vi "Post_Process_Raw_data.vi"(0 "Select Plug Ins":bool, 2 "Post processed Results folder":path, 3 "No dialogs":bool, 5 "Save results to":T1(ring)=enum."Original Results Filenames with _PP", 11 "Selected files":path[](array[path]), 12 "Current Results filenames":path[](array[path]), 13 "Results Plotter Rows":string[][](array[string])) -> (15 "Post processed Results folder Out":path)   [LabVIEW 2014]
uses:
  Anemometry Sub Vis/Controls/File_Selector_Type.ctl
  Anemometry Sub Vis/Controls/Setup.ctl
  Anemometry Sub Vis/Controls/Post_Process.ctl
  Anemometry Sub Vis/Controls/Save_Data.ctl
  Anemometry Sub Vis/Globals/Meas_global.vi
  Anemometry Sub Vis/Data_plotting_vis/Results_plotter_Global.vi
  Anemometry Sub Vis/Globals/Plug_in_data_global.vi
panel:
  out "Single Filename":string
  out "Files not found":i32
  out "Files not Found":path[](array[path])
  out "Checking":i32
  in  "Previous Choice":path
  in  "Search String":string
  in  "Boolean":bool
  in  "Pause Mode":enum16{"Continuous Running", "After Each File"}(ring)
  in  "At Dialog Prompt Post Process":T2=enum."All files listed in selected file"
  out "Files Processed":i32(slide) scale=0.0..1.0
  in  "stop":bool
  out "Files To Process":path[](array[path])
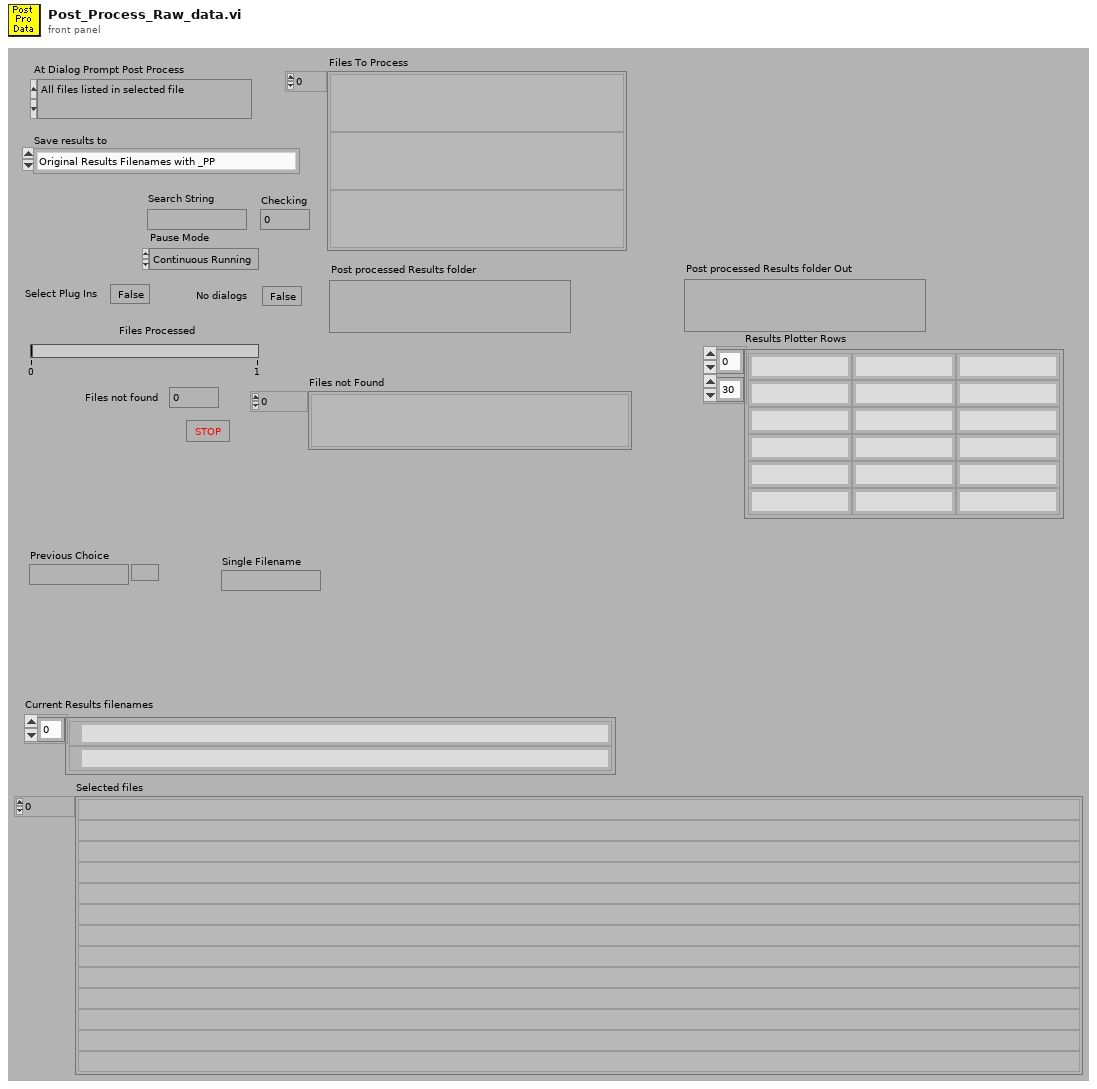
[diagram p1: front panel]
types:
  T1 = enum16{"A single file", "Original Results Filenames with _PP", "Current Results Filenames"}
  T2 = typedef "File_Selector_Type.ctl" = enum16{"The Selected File", "The Selected Folder", "Files containing the search string in the selected folder", "All files listed in selected file"}
  T3 = typedef "Setup.ctl" = enum16{"Run Program", "Show Setup", "Save Current Setup", "Setup Front Panel"}
  T4 = typedef "Save_Data.ctl" = enum16{"Save No Data", "Save Data"}
  T5 = typedef "Post_Process.ctl" = enum16{"Take New Data", "Post Process Raw Data File"}
  T6 = enum16{"Left Button", "Center Button", "Right Button", "Window Close"}
  T7 = typedef "Multi_Run_Status.ctl" = enum16{"Continue", "Jump to Next Point", "Jump to Next Row", "Jump To Fall Back", "Terminate Run"}
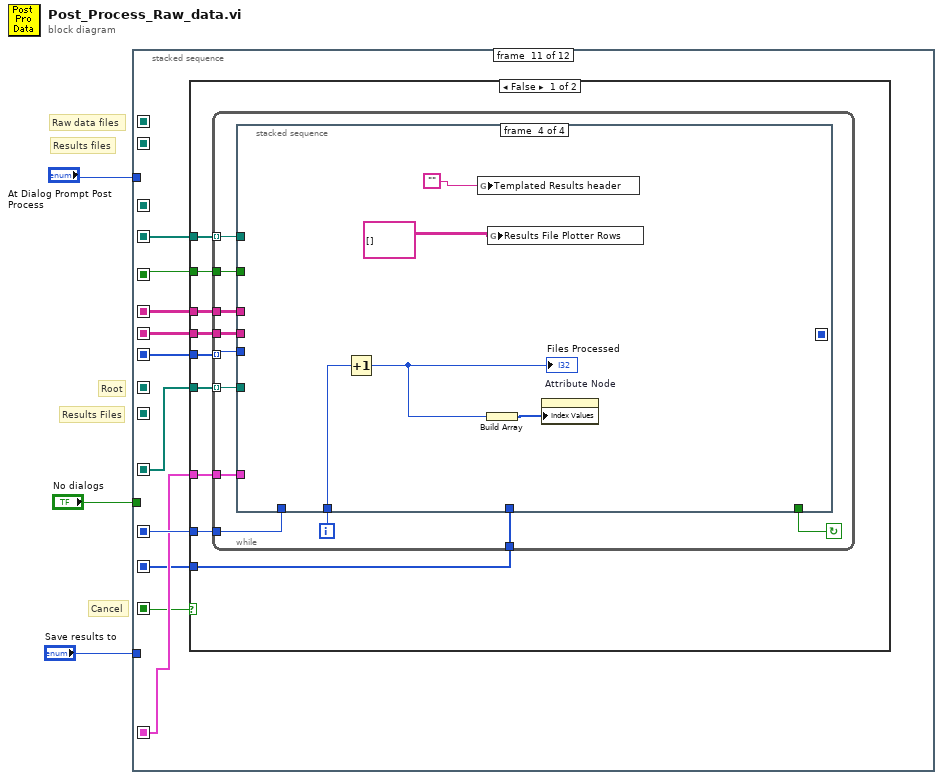
[diagram p0: block diagram]
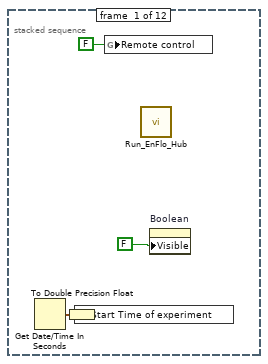
[diagram p2: hidden frame]
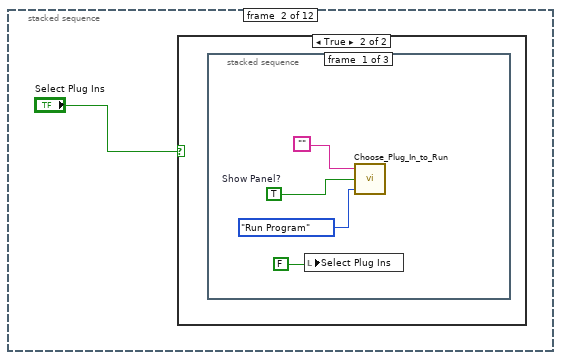
[diagram p3: hidden frame]
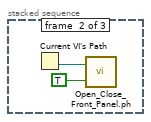
[diagram p5: hidden frame]
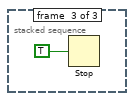
[diagram p6: hidden frame]
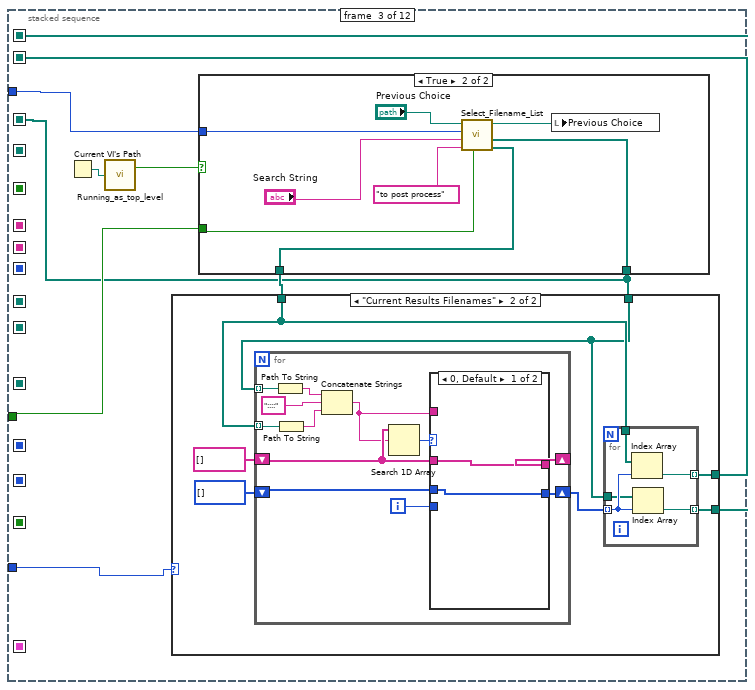
[diagram p7: hidden frame]
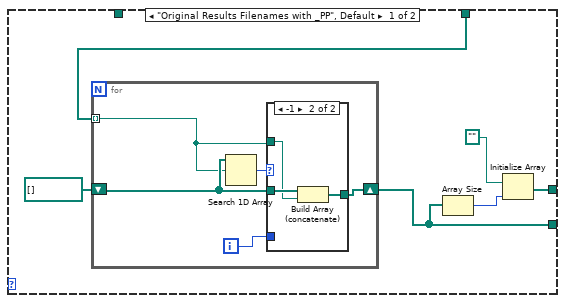
[diagram p8: hidden frame]
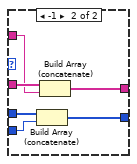
[diagram p10: hidden frame]
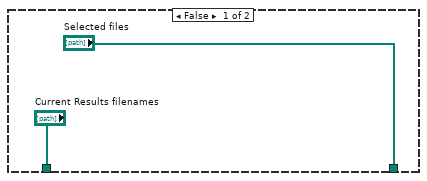
[diagram p11: hidden frame]
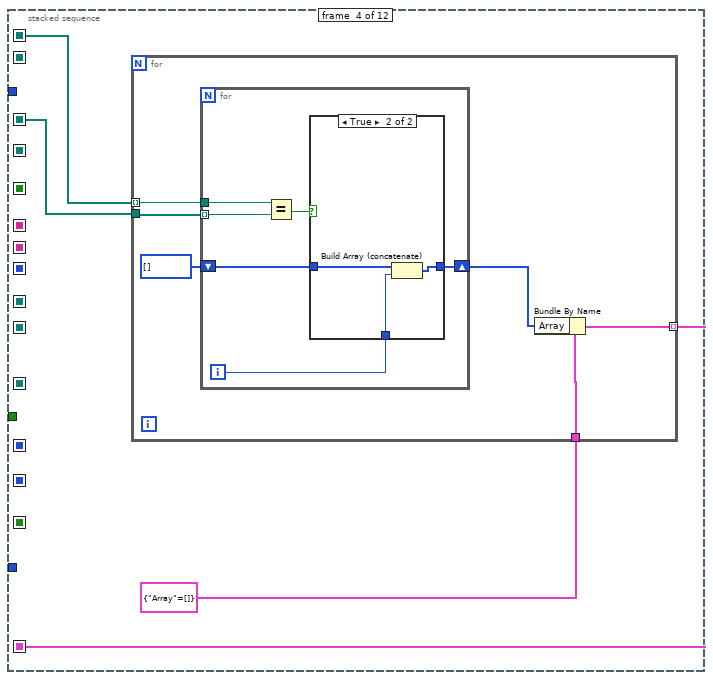
[diagram p12: hidden frame]
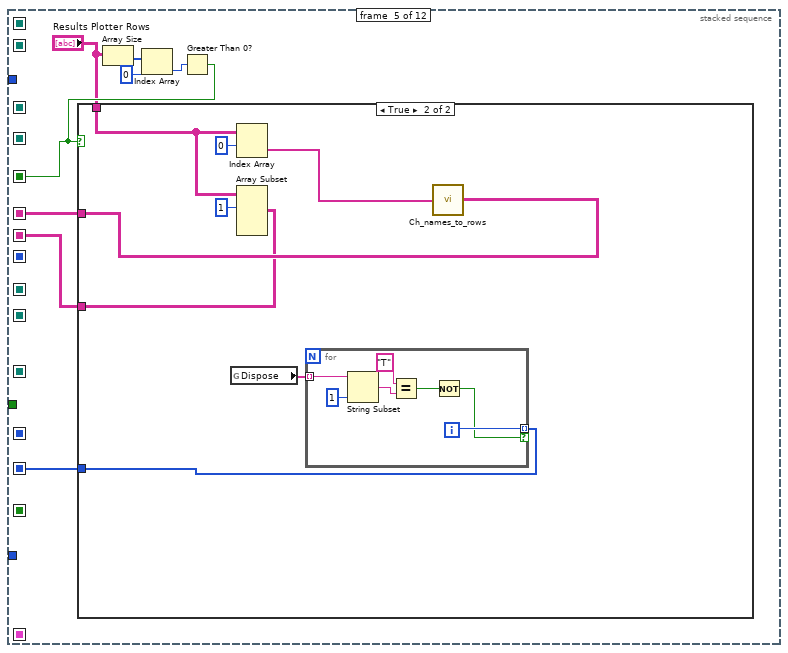
[diagram p14: hidden frame]
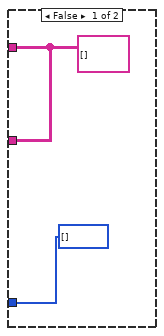
[diagram p15: hidden frame]
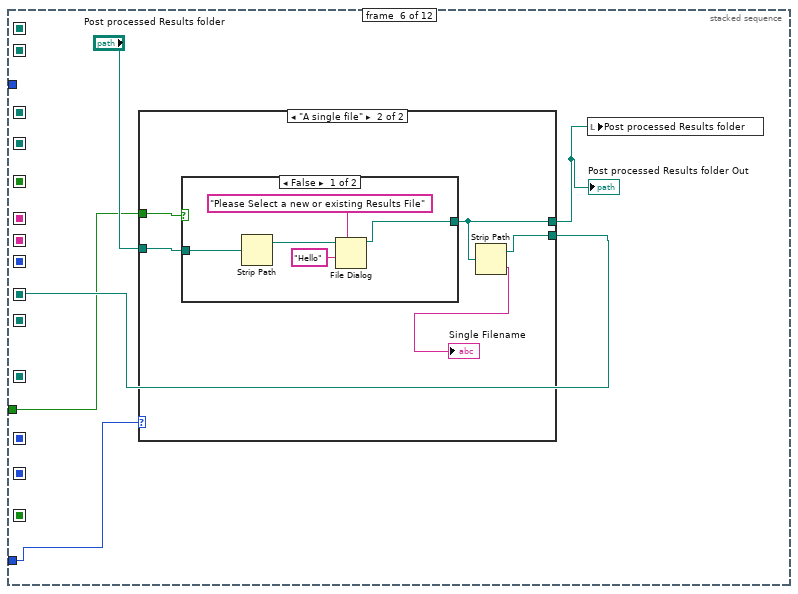
[diagram p16: hidden frame]
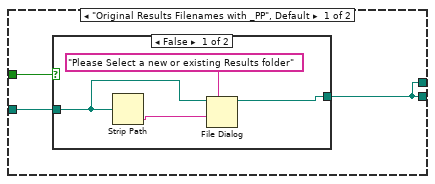
[diagram p17: hidden frame]
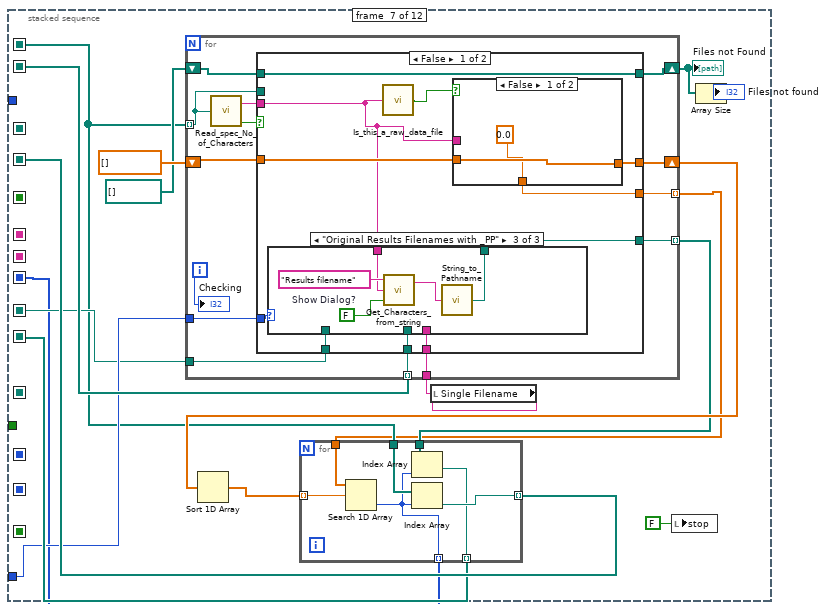
[diagram p20: hidden frame]
diagram:
  # "Cancel"
  # "Results files"
  # "Raw data files"
  # "Root"
  # "Results Files"
  n1 = stacked-sequence {
    seq-local: [_ _ _ _ _ _ w164 _ _ _ _ _] -> [_ _ _ _ _ _ _ _ _ w296 w311 _]
    seq-local: [_ _ _ _ _ _ _ _ _ w301 _ _] -> [_ _ _ _ _ _ _ _ _ _ w310 _]
    seq-local: [_ _ w18 _ _ _ _ _ _ _ _ _] -> [_ _ _ w84 _ _ w153 _ _ _ _ _]
    seq-local: [_ _ _ _ _ w131 _ _ _ _ _ _] -> [_ _ _ _ _ _ w156 w223 _ _ _ _]
    seq-local: [_ _ _ _ _ _ w162 _ _ _ _ _] -> [_ _ _ _ _ _ _ w226 _ _ _ _]
    seq-local: [_ _ _ _ _ _ _ w222 _ _ _ _] -> [_ _ _ _ _ _ _ _ w266 _ w309 w397]
    seq-local: [_ _ w19 _ _ _ _ _ _ _ _ _] -> [_ _ _ _ _ _ w158 _ _ _ _ _]
    seq-local: [_ _ _ _ w109 _ _ _ _ _ _ _] -> [_ _ _ _ _ _ _ _ _ _ w308 _]
    seq-local: [_ _ _ _ w108 _ _ _ _ _ _ _] -> [_ _ _ _ _ _ _ _ _ _ w305 _]
    seq-local: [_ _ _ _ w104 _ _ _ _ _ _ _] -> [_ _ _ _ _ _ _ _ _ _ w307 _]
    seq-local: [_ _ _ _ _ _ w154 _ _ _ _ _] -> [_ _ _ _ _ _ _ _ _ _ w306 _]
    seq-local: [_ _ _ w82 _ _ _ _ _ _ _ _] -> [_ _ _ _ _ _ _ _ _ _ w304 _]
    seq-local: [_ _ w16 _ _ _ _ _ _ _ _ _] -> [_ _ _ w85 _ _ _ _ _ _ _ _]
    seq-local: [_ _ _ _ _ _ _ _ w265 _ _ _] -> [_ _ _ _ _ _ _ _ _ _ w303 _]
    seq-local: [_ _ _ _ w102 _ _ _ _ _ _ _] -> [_ _ _ _ _ _ _ _ _ _ w302 _]
    tunnel: "At Dialog Prompt Post Process" -> [_ _ w24 _ _ _ _ _ _ _ _ _]
    tunnel: "No dialogs" -> [_ _ w23 _ _ w129 _ _ w267 _ _ _]
    tunnel: "Save results to" -> [_ _ w17 _ _ w128 w157 w225 _ _ _ _]
    frame #0 {
      n2 = Get Date/Time In Seconds() -> (seconds since 1Jan1904=w4:timestamp)
      n3 = To Double Precision Float(number=w4) -> (double precision float=w5:dbl)
      n4 = global write "Meas_global.vi" "Start Time of experiment"(w5) -> ()
      n5 = global write "Meas_global.vi" "Remote control"(FALSE ("Remote control")) -> ()
      n6 = call "Run_EnFlo_Hub.vi"() -> ()  [unwired: 8 out]
      n7 = property on="Boolean" class="Bool"("Visible"=FALSE ("Write Attribute")) -> ()  [unwired: 2 in, 2 out]
    }
    frame #1 {
      n8 = case shown="True" "Select Plug Ins" {
        frame False {
        }
        frame True {
          n9 = stacked-sequence {
            frame #0 {
              w12 = TRUE  # Show Panel?
              n10 = local write "Select Plug Ins"(FALSE ("Select Local ADAM Channels")) -> ()
              n11 = call "Choose_Plug_In_to_Run.vi"("setup"=Setup."Run Program", "Show Panel?"=w12, "Setup String In"="") -> ()  [unwired: 2 out]
            }
            frame #1 {
              n12 = Current VI's Path() -> (path=w14:path)
              n13 = call "Open_Close_Front_Panel.ph.vi"("Front Panel Window:Open"=TRUE, "VI path"=w14) -> ()  [unwired: 2 out]
            }
            frame #2 {
              n14 = Stop(stop? (T)=TRUE) -> ()
            }
          }
        }
      }
    }
    frame #2 {
      n15 = Current VI's Path() -> (path=w22:path)
      n16 = call "Running_as_top_level.vi"("Vi path name"=w22) -> ("Top Level"=w21:bool)  [unwired: 1 out]
      n17 = case shown="True" w21 {
        tunnel: w24 -> [_ w81]
        tunnel: w23 -> [_ w76]
        tunnel: ["Selected files" w75] -> w16
        tunnel: ["Current Results filenames" w74] -> w20
        frame False {
        }
        frame True {
          n18 = call "Select_Filename_List.vi"("No dialogs"=w76, "File Type"="to post process", "Search String"="Search String", "At Dialog Prompt Post Process"=w81, "Previous Choice"="Previous Choice") -> ("Current Results filenames"=w74:path[], "Selected files"=w75:path[], "Choosen path"=w77:path)  [unwired: 1 out]
          n19 = local write "Previous Choice"(w77) -> ()
        }
      }
      n20 = case shown="\"Current Results Filenames\"" w17 {
        tunnel: w16 -> [w30 w43]
        tunnel: w20 -> [_ w44]
        tunnel: [w26 w42] -> w19
        tunnel: [w28 w41] -> w18
        frame "Original Results Filenames with _PP", Default {
          n21 = for {
            shift-right: [w34] -> w28
            shift-left: path[] [] -> [w35]
            tunnel: w30 -> [w31] mode=indexing
            i -> [w32]
            n22 = Search 1D Array(1D array=w35, element=w31) -> (index of element=w33:i32)  [unwired: 1 out]
            n23 = case shown="-1" w33 {
              tunnel: w35 -> [w36 w39]
              tunnel: [w36 w38] -> w34
              tunnel: w31 -> [_ w37]
              tunnel: w32 -> [_ _]
              frame 0, Default {
              }
              frame -1 {
                n24 = Build Array (concatenate)(w39, w37) -> (w38:path[])
              }
            }
          }
          n25 = Array Size(array=w28) -> (size(s)=w27:i32)
          n26 = Initialize Array(path "", w27) -> (w26:path[])
        }
        frame "Current Results Filenames" {
          n27 = for {
            shift-right: [w62] -> _
            shift-left: string[] [] -> [w63]
            tunnel: w43 -> [w61] mode=indexing
            tunnel: w44 -> [w55] mode=indexing
            shift-right: [w57] -> w40
            shift-left: i32[] [] -> [w56]
            i -> [w58]
            n28 = Path To String(path=w61) -> (string=w60:string)
            n29 = Path To String(path=w55) -> (string=w54:string)
            n30 = Concatenate Strings(w60, "::::" ("string"), w54) -> (w53:string)
            n31 = Search 1D Array(1D array=w63, element=w53) -> (index of element=w52:i32)  [unwired: 1 out]
            n32 = case shown="0, Default" w52 {
              tunnel: w63 -> [w65 w71]
              tunnel: [w65 w70] -> w62
              tunnel: w53 -> [_ w67]
              tunnel: w58 -> [_ w66]
              tunnel: [w64 w69] -> w57
              tunnel: w56 -> [w64 w68]
              frame 0, Default {
              }
              frame -1 {
                n33 = Build Array (concatenate)(w68, w66) -> (w69:i32[])
                n34 = Build Array (concatenate)(w71, w67) -> (w70:string[])
              }
            }
          }
          n35 = for {
            tunnel: w40 -> [w51] mode=indexing
            tunnel: w44 -> [w50]
            tunnel: w43 -> [w49]
            tunnel: [w48] -> w42 mode=indexing
            tunnel: [w47] -> w41 mode=indexing
            n36 = Index Array(array=w50, index=w51) -> (element=w48:path)
            n37 = Index Array(array=w49, index=w51) -> (element=w47:path)
          }
        }
      }
    }
    frame #3 {
      n38 = for {
        tunnel: w85 -> [w90]
        tunnel: w84 -> [w91] mode=indexing
        tunnel: cluster{"Array":i64[]} {"Array"=[]} ("Cluster") -> [w88]
        tunnel: [w86] -> w82 mode=indexing
        n39 = for {
          tunnel: w91 -> [w97]
          tunnel: w90 -> [w96] mode=indexing
          shift-right: [w93] -> w87
          shift-left: i32[] [] -> [w94]
          i -> [w92]
          n40 = Equal?(x=w97, y=w96) -> (x = y?=w95:bool)
          n41 = case shown="True" w95 {
            tunnel: w94 -> [w98 w101]
            tunnel: [w98 w100] -> w93
            tunnel: w92 -> [_ w99]
            frame False {
            }
            frame True {
              n42 = Build Array (concatenate)(w101, w99) -> (w100:i32[])
            }
          }
        }
        n43 = Bundle By Name(cluster=w88, "Array"=w87) -> (w86:cluster{"Array":i64[]})
      }
    }
    frame #4 {
      n44 = Array Size(array="Results Plotter Rows") -> (size(s)=w107:i32[])
      n45 = Index Array(array=w107, index=0) -> (element=w105:i32)
      n46 = Greater Than 0?(x=w105) -> (x > 0?=w104:bool)
      n47 = case shown="True" w104 {
        tunnel: [w111 w119] -> w109
        tunnel: [w111 w114] -> w108
        tunnel: "Results Plotter Rows" -> [_ w117]
        tunnel: [i32[] [] w112] -> w102
        frame False {
          w111 = string[][] [] ("3 Row names")
        }
        frame True {
          n48 = global read "Results_plotter_Global.vi" "Dispose"() -> (w113:string[])
          n49 = Index Array(array=w117, index (row)=0 ("index")) -> (element=w115:string[])  [unwired: 1 in]
          n50 = Array Subset(array=w117, index (row)=1 ("index")) -> (w114:string[][])  [unwired: 3 in]
          n51 = for {
            tunnel: w113 -> [w123] mode=indexing
            tunnel: [w122] -> w112 mode=indexing if=w120
            i -> [w122]
            n52 = String Subset(string=w123, length (rest)=1 ("length (rest)")) -> (substring=w125:string)  [unwired: 1 out]
            n53 = Equal?(x="T", y=w125) -> (x = y?=w121:bool)
            n54 = Not(x=w121) -> (.not. x?=w120:bool)
          }
          n55 = call "Ch_names_to_rows.vi"("Channel Names"=w115) -> ("3 Row names"=w119:string[][])
        }
      }
    }
    frame #5 {
      n56 = case shown="\"A single file\"" w128 {
        tunnel: [w132 w141] -> w131
        tunnel: "Post processed Results folder" -> [w134 w144]
        tunnel: w129 -> [w133 w143]
        tunnel: [w132 w142] -> w127
        frame "Original Results Filenames with _PP", Default {
          n57 = case shown="False" w133 {
            tunnel: [w138 w139] -> w132
            tunnel: w134 -> [w135 w139]
            frame False {
              n58 = Strip Path(path=w135) -> (name=w136:string)  [unwired: 1 out]
              n59 = File Dialog(7:"Please Select a new or existing Results folder" ("prompt"), 9:w136, 11:w135) -> (3:w138:path)  [unwired: 1 in, 6 out]
            }
            frame True {
            }
          }
        }
        frame "A single file" {
          n60 = case shown="False" w143 {
            tunnel: w144 -> [w148 w150]
            tunnel: [w147 w150] -> w142
            frame False {
              n61 = Strip Path(path=w148) -> (stripped path=w146:path)  [unwired: 1 out]
              n62 = File Dialog(7:"Please Select a new or existing Results File" ("prompt"), 9:"Hello" ("default name"), 11:w146) -> (3:w147:path)  [unwired: 1 in, 6 out]
            }
            frame True {
            }
          }
          n63 = Strip Path(path=w142) -> (stripped path=w141:path, name=→"Single Filename":string)
        }
      }
      "Post processed Results folder Out" <- w127
      n64 = local write "Post processed Results folder"(w127) -> ()
    }
    frame #6 {
      n65 = local read "Single Filename"() -> (w155:string)
      n66 = for {
        tunnel: w153 -> [w183] mode=indexing
        shift-right: [w187] -> w167
        shift-left: dbl[] [] -> [w188]
        shift-right: [w184] -> w160
        shift-left: path[] [] -> [w185]
        tunnel: w158 -> [w180] mode=indexing
        tunnel: w157 -> [w179]
        tunnel: w156 -> [w178]
        tunnel: w155 -> [w177]
        tunnel: [w176] -> w152 mode=indexing
        tunnel: [w175] -> w151 mode=indexing
        i -> [w186]
        n67 = call "Read_spec_No_of_Characters.vi"("Filename"=w183) -> ("character string"=w182:string, "Error?"=w181:bool)
        n68 = case shown="False" w181 {
          tunnel: w188 -> [w199 w221]
          tunnel: [w198 w221] -> w187
          tunnel: w183 -> [_ w219]
          tunnel: w185 -> [w196 w220]
          tunnel: [w196 w218] -> w184
          tunnel: w182 -> [w195 _]
          tunnel: w180 -> [w193 w217]
          tunnel: w179 -> [w194 _]
          tunnel: w178 -> [w192 _]
          tunnel: w177 -> [w191 _]
          tunnel: [w190 w217] -> w176
          tunnel: [w189 0.0 ("Value")] -> w175
          frame False {
            n69 = case shown="\"Original Results Filenames with _PP\"" w194 {
              tunnel: [w202 w203 w206] -> w190
              tunnel: w195 -> [_ _ w204]
              tunnel: w193 -> [_ w203 _]
              tunnel: w192 -> [w201 _ _]
              tunnel: w191 -> [w200 _ _]
              frame "A single file" {
                n70 = Build Path(base path=w201, name or relative path=w200) -> (appended path=w202:path)
              }
              frame "Current Results Filenames" {
              }
              frame "Original Results Filenames with _PP" {
                w207 = FALSE  # Show Dialog?
                n71 = call "Get_Characters_from_string.vi"("Show Dialog?"=w207, "Input string"=w204, "Variable name"="Results filename") -> ("Value"=w205:string)  [unwired: 1 out]
                n72 = call "String_to_Pathname.vi"("Input String"=w205) -> ("path"=w206:path)
              }
            }
            n73 = call "Is_this_a_raw_data_file.vi"("character string"=w195) -> ("Raw Dat File?"=w197:bool)  [unwired: 2 out]
            n74 = case shown="False" w197 {
              tunnel: w199 -> [w210 w212]
              tunnel: [w210 w215] -> w198
              tunnel: w195 -> [_ w213]
              tunnel: [0.0 ("Value") w211] -> w189
              frame False {
              }
              frame True {
                n75 = call "Get_value_from_string.vi"("Input string"=w213, "Variable name"="Seconds since 1/1/04") -> ("Value"=w211:dbl)  [unwired: 1 in, 1 out]
                n76 = Build Array (concatenate)(w212, w211) -> (w215:dbl[])
              }
            }
          }
          frame True {
            n77 = Build Array (concatenate)(w220, w219) -> (w218:path[])
          }
        }
        "Checking" <- w186
      }
      "Files not Found" <- w160
      n78 = Sort 1D Array(array=w167) -> (sorted array=w166:dbl[])
      n79 = for {
        tunnel: w151 -> [w174]
        tunnel: w166 -> [w173] mode=indexing
        tunnel: w153 -> [w172]
        tunnel: [w171] -> w164 mode=indexing
        tunnel: w152 -> [w170]
        tunnel: [w169] -> w162 mode=indexing
        tunnel: [w168] -> w154 mode=indexing
        n80 = Search 1D Array(1D array=w174, element=w173) -> (index of element=w168:i32)  [unwired: 1 out]
        n81 = Index Array(array=w170, index=w168) -> (element=w169:path)
        n82 = Index Array(array=w172, index=w168) -> (element=w171:path)
      }
      n83 = local write "stop"(FALSE ("stop")) -> ()
      n84 = Array Size(array=w160) -> (size(s)=→"Files not found":i32)
    }
    frame #7 {
      n85 = case shown="\"Original Results Filenames with _PP\"" w225 {
        tunnel: [FALSE TRUE] -> w224
        tunnel: w225 -> [_ _]
        frame "A single file", Default {
        }
        frame "Original Results Filenames with _PP" {
        }
      }
      n86 = for {
        tunnel: w226 -> [w260] mode=indexing
        tunnel: w224 -> [w232]
        tunnel: w223 -> [w231]
        tunnel: [w229] -> w222 mode=indexing
        w245 = "_" ("Replace with")
        n87 = Strip Path(path=w260) -> (name=w233:string)  [unwired: 1 out]
        n88 = Concatenate Strings("[" ("Substring"), ":", "/", "\\\\", "|", "?", ">", "<", "*", "\"", "]" ("Substring")) -> (w248:string)
        n89 = call <vilib>:"Trim Whitespace.vi"("string"=w233) -> ("trimmed string"=w247:string)  [unwired: 1 in]
        n90 = call "Add_filename_suffix.vi"("Filename"=w247) -> ("Original Suffix"=w237:string, "Base name"=w246:string)  [unwired: 1 in, 2 out]
        n91 = call "Replace_Character.vi"("Replace with"=w245, "Input String"=w246, "Search For"=w248) -> ("Output string"=w241:string)  [unwired: 1 out]
        n92 = call "Replace_Character.vi"("Replace with"="_", "Input String"=w241, "Search For"=" ") -> ("Output string"=w242:string)  [unwired: 1 out]
        n93 = case shown="False" w232 {
          tunnel: [w261 w263] -> w244
          tunnel: w242 -> [w261 w262]
          frame False {
          }
          frame True {
            n94 = Concatenate Strings(w262, "_pp" ("Substring")) -> (w263:string)
          }
        }
        n95 = Empty String/Path?(string/path=w237) -> (empty?=w238:bool)
        n96 = Select(t=".xls", s=w238, f=w237) -> (s? t:f=w236:string)
        n97 = call "Replace_Character.vi"("Replace with"=w245, "Input String"=w244, "Search For"="__") -> ("Output string"=w235:string)  [unwired: 1 out]
        n98 = Concatenate Strings(w235, w236) -> (w230:string)
        n99 = Build Path(base path=w231, name or relative path=w230) -> (appended path=w229:path)
      }
    }
    frame #8 {
      n100 = case shown="False" w267 {
        tunnel: w266 -> [w271 w291]
        tunnel: [w268 FALSE ("stop? (T)")] -> w265
        frame False {
          n101 = Path To String(path=w271) -> (string=w270:string[])
          n102 = call "Analyse_string_array.vi"("String array"=w270) -> ("Unique strings"=w269:string[])  [unwired: 2 out]
          n103 = for {
            tunnel: w269 -> [w274] mode=indexing
            tunnel: [w273] -> w268
            stop <- w273 stop-if-true
            n104 = String To Path(string=w274) -> (path=w272:path)
            n105 = call "Does_file_exist_(simple).vi"("Pathname"=w272) -> ("exists?"=w275:bool)
            n106 = call "Create_directory_path.vi"("Path name"=w272) -> ()  [unwired: 1 in, 2 out]
            n107 = case shown="True" w275 {
              tunnel: w272 -> [_ w280]
              tunnel: [FALSE ("stop? (T)") w279] -> w273
              frame False {
              }
              frame True {
                n108 = Format Into String(format string="%s\nAlready exists. ", w280) -> (resulting string=w283:string)  [unwired: 2 in, 1 out]
                n109 = call <vilib>:"Three Button Dialog.vi"("Allow user to close window? (TRUE)"=FALSE, "Center Button Text (\"No\")"="Append" ("Center Button Text (\"No\")"), "Left Button Text (\"Yes\")"="Overwrite" ("Left Button Text (\"Yes\")"), "message"=w283) -> ("Which Button?"=w281:T6)  [unwired: 7 in]
                n110 = case shown="\"Center Button\"" w281 {
                  tunnel: w280 -> [w286 _ _ _]
                  tunnel: [FALSE ("stop? (T)") FALSE ("stop? (T)") TRUE ("stop? (T)") FALSE ("stop? (T)")] -> w279
                  frame "Left Button" {
                    n111 = Delete(path (use dialog)=w286) -> ()  [unwired: 4 in, 3 out]
                  }
                  frame "Center Button" {
                  }
                  frame "Right Button" {
                  }
                  frame "Window Close" {
                  }
                }
              }
            }
          }
        }
        frame True {
          n112 = Path To String(path=w291) -> (string=w292:string[])
          n113 = call "Analyse_string_array.vi"("String array"=w292) -> ("Unique strings"=w290:string[])  [unwired: 2 out]
          n114 = for {
            tunnel: w290 -> [w295] mode=indexing
            n115 = String To Path(string=w295) -> (path=w294:path)
            n116 = call "Create_directory_path.vi"("Path name"=w294) -> ()  [unwired: 1 in, 2 out]
          }
        }
      }
    }
    frame #9 {
      w297 = 0 ("Files Processed")
      n117 = Array Size(array=w296) -> (size(s)=w301:i32)
      n118 = Array Size(array=w296) -> (size(s)=w299:i32)
      n119 = property on="Files Processed" class="Slide (strict)"("Scale.Range:Minimum"=0.0 ("Write Attribute"), "Scale.Range:Maximum"=w299) -> ()  [unwired: 2 in, 2 out]
      n120 = local write "Files Processed"(w297) -> ()
      n121 = Build Array(w297) -> (w298:i32[])
      n122 = property on="Attribute Node" class="Arr (strict)"("Index Values"=w298) -> ()  [unwired: 2 in, 2 out]
      "Files To Process" <- w296
    }
    frame #10 {
      n123 = case shown="False" w303 {
        tunnel: w311 -> [w320 _]
        tunnel: w310 -> [w319 _]
        tunnel: w309 -> [w318 _]
        tunnel: w308 -> [w317 _]
        tunnel: w307 -> [w316 _]
        tunnel: w306 -> [w315 _]
        tunnel: w305 -> [w314 _]
        tunnel: w304 -> [w313 _]
        tunnel: w302 -> [w312 _]
        frame False {
          n124 = while {
            tunnel: w318 -> [w327] mode=indexing
            tunnel: w319 -> [w330]
            tunnel: w320 -> [w331] mode=indexing
            tunnel: w317 -> [w326]
            tunnel: w315 -> [w323] mode=indexing
            tunnel: w316 -> [w325]
            tunnel: w314 -> [w324]
            tunnel: w313 -> [w322]
            tunnel: w312 -> [w321]
            i -> [w329]
            stop <- w328 continue-if-true
            n125 = stacked-sequence {
              seq-local: [_ w364 _ _] -> [_ _ w368 _]
              tunnel: w327 -> [_ w366 _ _]
              tunnel: w331 -> [_ w365 _ _]
              tunnel: w330 -> [_ _ w370 _]
              tunnel: w329 -> [_ _ w369 w394]
              tunnel: [_ _ w367 _] -> w328
              tunnel: w326 -> [w342 _ _ _]
              tunnel: w325 -> [w341 _ _ _]
              tunnel: w324 -> [w337 _ _ _]
              tunnel: w323 -> [w338 _ _ _]
              tunnel: w322 -> [w339 _ _ _]
              tunnel: w321 -> [w333 _ _ _]
              frame #0 {
                n126 = Index Array(array=w339, index=w338) -> (element=w336:cluster{"Array":i64[]})
                n127 = Unbundle By Name(w336) -> ("Array"=w335:i64[])
                n128 = for {
                  tunnel: w337 -> [w345]
                  tunnel: w335 -> [w344] mode=indexing
                  tunnel: [w343] -> w334 mode=indexing
                  n129 = Index Array(array=w345, index (row)=w344) -> (element=w343:string[])  [unwired: 1 in]
                }
                n130 = case shown="True" w341 {
                  tunnel: w342 -> [_ w353]
                  tunnel: w334 -> [_ w348]
                  tunnel: ["" w352] -> w340
                  tunnel: w333 -> [_ w351]
                  tunnel: [string[][] [] ("3 Row names") w348] -> w332
                  frame False {
                  }
                  frame True {
                    n131 = Build Array (concatenate)(w353, w348) -> (w350:string[][])
                    n132 = for {
                      tunnel: w351 -> [w357]
                      tunnel: w350 -> [w356] mode=indexing
                      tunnel: [w355] -> w349 mode=indexing
                      n133 = for {
                        tunnel: w357 -> [w360] mode=indexing
                        tunnel: w356 -> [w359]
                        tunnel: [w358] -> w355 mode=indexing
                        n134 = Index Array(array=w359, index=w360) -> (element=w358:string)
                      }
                    }
                    n135 = Array To Spreadsheet String(array=w349, 3:"%s" ("format string")) -> (spreadsheet string=w352:string)  [unwired: 1 out]
                  }
                }
                n136 = global write "Plug_in_data_global.vi" "Results File Plotter Rows"(w332) -> ()
                n137 = global write "Plug_in_data_global.vi" "Templated Results header"(w340) -> ()
              }
              frame #1 {
                n138 = call "Measurement.vi"("setup"=Setup."Run Program", "Post Process"=Post_Process."Post Process Raw Data File", "File"=Save_Data."Save Data", "Results file"=w366, "Raw data file"=w365) -> ("Status Out"=w364:T7)  [unwired: 2 in, 12 out]
              }
              frame #2 {
                n139 = Increment(x=w369) -> (x+1=w372:i32)
                n140 = Less?(x=w372, y=w370) -> (x < y?=w371:bool)
                n141 = while {
                  shift-left: _ -> [w378]
                  shift-right: [w379] -> _
                  tunnel: [w381] -> w367
                  tunnel: w368 -> [w382]
                  tunnel: w371 -> [w374]
                  stop <- w377 continue-if-true
                  n142 = case shown="\"After Each File\"" "Pause Mode" {
                    tunnel: [TRUE "Boolean"] -> w376
                    tunnel: w378 -> [_ w387]
                    frame "Continuous Running" {
                    }
                    frame "After Each File" {
                      n143 = Select(t=u32 500 ("milliseconds to wait"), s=w387, f=u32 100) -> (s? t:f=w384:u32)
                      n144 = property on="Boolean" class="Bool"("Visible"=w387, "Key Focus"=w387) -> ()  [unwired: 2 in, 2 out]
                      n145 = Wait (ms)(milliseconds to wait=w384) -> ()  [unwired: 1 out]
                    }
                  }
                  n146 = Compound Arithmetic op=AND(invert w376, invert "stop", w374) -> (w377:bool)
                  n147 = Compound Arithmetic op=AND(w376, invert "stop", w374) -> (w373:bool)
                  n148 = case shown="\"Terminate Run\"" w382 {
                    tunnel: [w389 FALSE] -> w381
                    tunnel: w373 -> [w389 _]
                    frame "Continue", Default {
                    }
                    frame "Terminate Run" {
                    }
                  }
                  n149 = Not(x=w378) -> (.not. x?=w379:bool)
                }
              }
              frame #3 {
                n150 = Increment(x=w394) -> (x+1=w393:i32)
                "Files Processed" <- w393
                n151 = global write "Plug_in_data_global.vi" "Templated Results header"("") -> ()
                n152 = Build Array(w393) -> (w395:i32[])
                n153 = global write "Plug_in_data_global.vi" "Results File Plotter Rows"(string[][] [] ("Results File Plotter Rows")) -> ()
                n154 = property on="Attribute Node" class="Arr (strict)"("Index Values"=w395) -> ()  [unwired: 2 in, 2 out]
              }
            }
          }
        }
        frame True {
        }
      }
    }
    frame #11 {
      n155 = Path To String(path=w397) -> (string=w399:string[])
      n156 = call "Analyse_string_array.vi"("String array"=w399) -> ("Unique strings"=w398:string[])  [unwired: 2 out]
      n157 = String To Path(string=w398) -> (path=w396:path[])
      n158 = for {
        tunnel: w396 -> [w403] mode=indexing
        w404 = FALSE  # Lock File
        n159 = call "Lock_File.vi"("Lock File"=w404, "path"=w403) -> ()  [unwired: 1 in, 3 out]
      }
      n160 = Build Array(0) -> (w401:i32[])
      n161 = property on="Boolean" class="Bool"("Visible"=FALSE ("Write Attribute")) -> ()  [unwired: 2 in, 2 out]
      n162 = property on="Attribute Node" class="Arr (strict)"("Index Values"=w401) -> ()  [unwired: 2 in, 2 out]
    }
  }
